vi "Remove Wheels from Steering Frame.vi"   [LabVIEW 2017, in "NI_Robotics_Steering Frame.lvclass"]
doc: "Removes the wheel or wheels you specify from <B>steering frame in</B>. You must manually select the polymorphic instance to use."
uses:
  <vilib>/robotics/Steering/Steering Frame/NI_Robotics_Steering Frame.lvclass
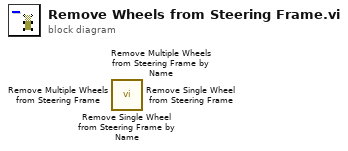
[diagram p0: block diagram]
diagram:
  n1 = call <vilib>:"Remove Single Wheel from Steering Frame by Name.vi"() -> ()  [unwired: 5 in, 7 out]
  n2 = call <vilib>:"Remove Multiple Wheels from Steering Frame by Name.vi"() -> ()  [unwired: 5 in, 7 out]
  n3 = call <vilib>:"Remove Multiple Wheels from Steering Frame.vi"() -> ()  [unwired: 5 in, 7 out]
  n4 = call <vilib>:"Remove Single Wheel from Steering Frame.vi"() -> ()  [unwired: 5 in, 7 out]
